vi "Autosort Is Name Unique.vi"(8 "error in (no error)":errorcluster, 11 "Name":string) -> (0 "error out":errorcluster, 3 "Is Name Unique?":bool)   [LabVIEW 2016]
uses:
  Autosort Parameters Set.vi
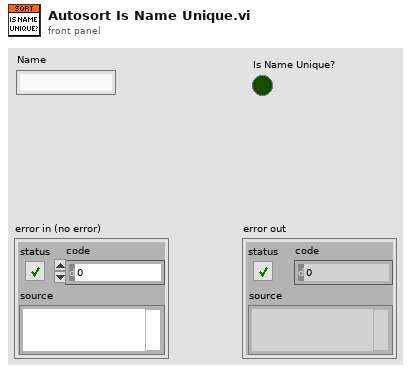
[diagram p1: front panel]
types:
  T1 = typedef "Autosort Parameters.ctl" = cluster{"Name":string, "Min Vel":dbl, "Trigger Ch":i32, "MaxVel":dbl, "Width":i32, "Pre Impuls":i32, "Post Impuls":i32, "Pitch":dbl, "Other Trigger":bool, "Cross Corr":bool}
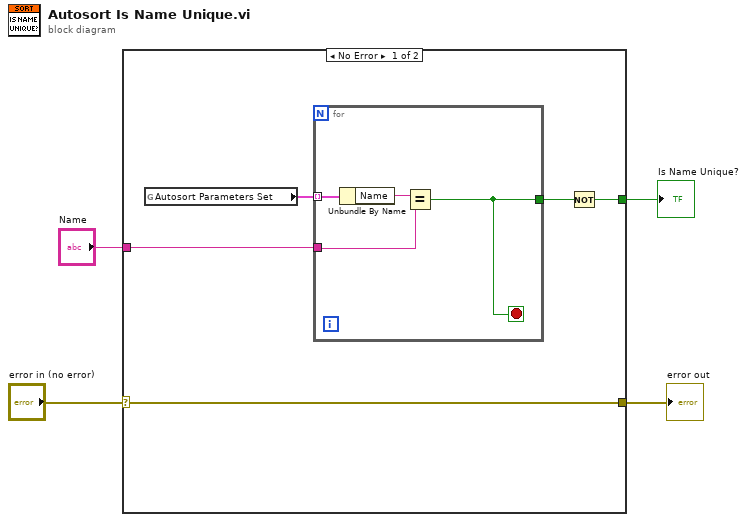
[diagram p0: block diagram]
diagram:
  n1 = case shown="No Error" "error in (no error)" {
    selector: "error in (no error)" -> [w5 w14]
    tunnel: "Name" -> [w8 _]
    tunnel: [w6 _] -> w3
    tunnel: [w5 w14] -> w1
    frame No Error {
      n2 = global read "Autosort Parameters Set.vi" "Autosort Parameters Set"() -> (w9:T1[])
      n3 = for {
        tunnel: w9 -> [w13] mode=indexing
        tunnel: w8 -> [w11]
        tunnel: [w10] -> w7
        stop <- w10 stop-if-true
        n4 = Unbundle By Name(w13) -> ("Name"=w12:string)
        n5 = Equal?(x=w12, y=w11) -> (x = y?=w10:bool)
      }
      n6 = Not(x=w7) -> (.not. x?=w6:bool)
    }
    frame Error {
    }
  }
  "error out" <- w1
  "Is Name Unique?" <- w3
